vi "setAll.vi"(8 "error in (no error)":errorcluster, 10 "MonoSetup":T4, 11 "MonoClientCommunicator in":refnum<class "MonoClientCommunicator.lvclass">) -> (0 "error out":errorcluster, 2 "ack":T5, 3 "MonoClientCommunicator out":refnum<class "MonoClientCommunicator.lvclass">)   [LabVIEW 2016, in "MonoClientCommunicator.lvclass"]
uses:
  MonoClientCommunicator.lvclass
  Typedefs/AckType.ctl
  Typedefs/wavelength.ctl
  Typedefs/slitWidth.ctl
  Typedefs/GratingType.ctl
  Typedefs/MonoCommand.ctl
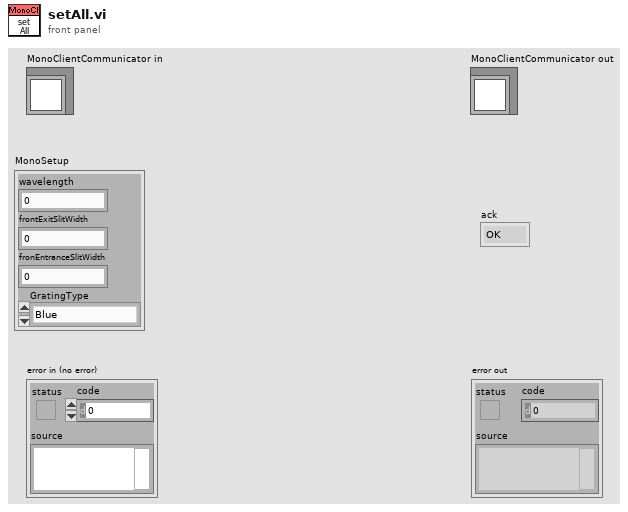
[diagram p1: front panel]
types:
  T1 = typedef "wavelength.ctl" = dbl
  T2 = typedef "slitWidth.ctl" = dbl
  T3 = typedef "GratingType.ctl" = enum16{"Blue", "Red", "Mirror"}
  T4 = cluster{"wavelength":T1, "frontExitSlitWidth":T2, "fronEntranceSlitWidth":T2, "GratingType":T3}
  T5 = typedef "AckType.ctl" = enum16{"OK", "OutOfRange", "Unknown", "Busy", "Rejected"}
  T6 = typedef "MonoCommand.ctl" = enum16{"getGrating", "getFrontEntranceSlitPosition", "getFrontExitSlitPosition", "getWavelength", "setWavelength", "setGrating", "setFrontEntranceSlitPosition", "setFrontExitSlitPosition", "calibrateWavelength", "getStatus", "Unknown", "reset", "setAll"}
  T7 = typedef "publishers.ctl" = enum16{"Wavelength", "Grating", "FrontEntranceSlitPosition", "FrontExitSlitPosition", "SoftwareStatus", "MonochromatorId", "Ack"}
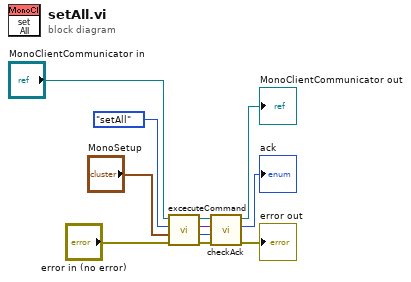
[diagram p0: block diagram]
diagram:
  n1 = call "excecuteCommand.vi"("error in (no error)"="error in (no error)", "input"="MonoSetup", "MonoCommand"=MonoCommand."setAll", "MonoClientCommunicator in"="MonoClientCommunicator in") -> ("error out"=w11:errorcluster, "parameter"=w8:T7, "value"=w9:variant, "MonoClientCommunicator out"=w10:refnum<class "MonoClientCommunicator.lvclass">)  [unwired: 4 in]
  n2 = call "checkAck.vi"("error in (no error)"=w11, "type"=w8, "value"=w9, "MonoClientCommunicator in"=w10) -> ("error out"=→"error out":errorcluster, "ack"=→"ack":T5, "MonoClientCommunicator out"=→"MonoClientCommunicator out":refnum<class "MonoClientCommunicator.lvclass">)  [unwired: 5 in]
